vi "Neg Binomial Random.vi"(6 "seed":i32=-1, 7 "reset":bool, 9 "p":dbl=0.5, 10 "x":dbl=5.0, 11 "samples":i32=128) -> (0 "error":i32, 3 "neg binomial random data":i32[](array[numeric]))   [LabVIEW 2010, in "NI_Gmath.lvlib"]
doc: "Generates random values from a variate X, where X describes the selected distribution type. You must manually select the polymorphic instance to use."
uses:
  NI_Gmath.lvlib
panel:
  # "Neg Binomial Random"
  # "successes"
  # "probability"
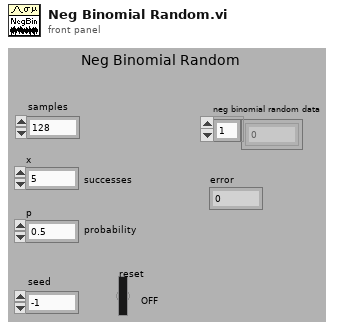
[diagram p1: front panel]
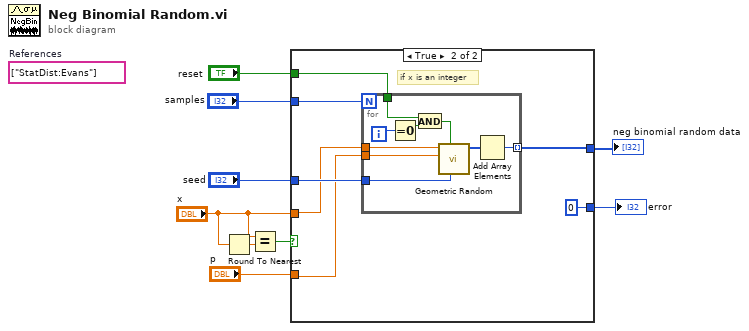
[diagram p0: block diagram]
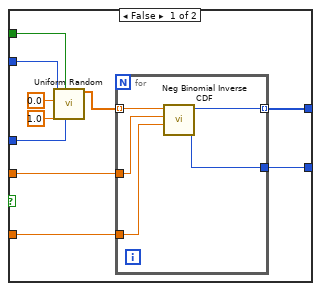
[diagram p2: hidden frame]
diagram:
  (unwired) string[] ["StatDist:Evans"]  # References
  n1 = Round To Nearest(number="x") -> (nearest integer value=w3:dbl)
  n2 = Equal?(x="x", y=w3) -> (x = y?=w1:bool)
  n3 = case shown="True" w1 {
    tunnel: "p" -> [w19 w28]
    tunnel: [w18 w27] -> w8
    tunnel: [w17 0 ("error")] -> w7
    tunnel: "samples" -> [w16 w25]
    tunnel: "x" -> [w12 w29]
    tunnel: "seed" -> [w11 w30]
    tunnel: "reset" -> [w10 w31]
    frame False {
      n4 = call "Uniform Random.vi"("seed"=w11, "reset"=w10, "xmax"=1.0, "xmin"=0.0, "samples"=w16) -> ("uniform random data"=w13:dbl[])  [unwired: 5 in, 1 out]
      n5 = for {
        tunnel: w13 -> [w24] mode=indexing
        tunnel: w12 -> [w21]
        tunnel: w19 -> [w20]
        tunnel: [w23] -> w18 mode=indexing
        tunnel: [w22] -> w17
        n6 = call "Neg Binomial Inverse CDF.vi"("p"=w20, "x"=w21, "cdf(y)"=w24) -> ("error"=w22:i32, "y"=w23:i32)  [unwired: 7 in]
      }
    }
    frame True {
      # "if x is an integer"
      n7 = for {
        N: w25 -> [_]
        tunnel: w31 -> [w38]
        tunnel: w30 -> [w36]
        tunnel: w29 -> [w35]
        tunnel: w28 -> [w34]
        tunnel: [w32] -> w27 mode=indexing
        i -> [w40]
        n8 = Equal To 0?(x=w40) -> (x = 0?=w39:bool)
        n9 = And(x=w38, y=w39) -> (x .and. y?=w37:bool)
        n10 = call "Geometric Random.vi"("seed"=w36, "reset"=w37, "p"=w34, "samples"=w35) -> ("geometric random data"=w33:i32[])  [unwired: 6 in, 1 out]
        n11 = Add Array Elements(numeric array=w33) -> (sum=w32:i32)
      }
    }
  }
  "error" <- w7
  "neg binomial random data" <- w8
